vi "Control System.vi"(0 "VISA resource name":refnum<visa-resource-name>, 1 "Enable Zero Correct (F: Disable)":bool, 2 "Autoranging Speed (0: Fast)":i32(ring) items=["Fast", "Normal"], 5 "Enable Line Synchronization (T: Enable)":bool=TRUE, 7 "Enable A/D Hardware Limit (T: Enable)":bool=TRUE, 9 "Enable Humidity Readings (F: Disable)":bool, 11 "error in (no error)":errorcluster) -> (4 "VISA resource name out":refnum<visa-resource-name>, 15 "error out":errorcluster)   [LabVIEW 2019, in "Keithley 6517.lvlib"]
doc: "Controls the system line synchronization, A/D hardware limit, humidity readings, zero correction and autoranging.\n\nNote:\nRequires a separate scanner card. According to the manual 6521 or 6522, 7001 and 7002 can be used with this model. If the scanner card is not used the error -241, \"Hardware missing\" will be generated.\n\nThis VI is <B>NOT</B> compatible with model <B>6514</B>."
uses:
  Keithley 6517.lvlib
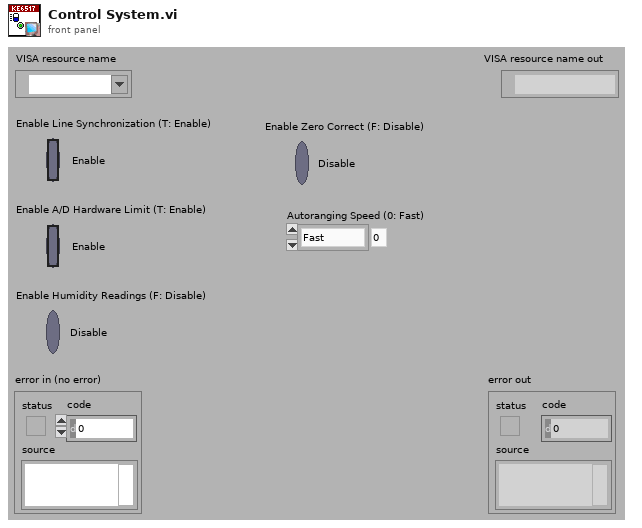
[diagram p1: front panel]
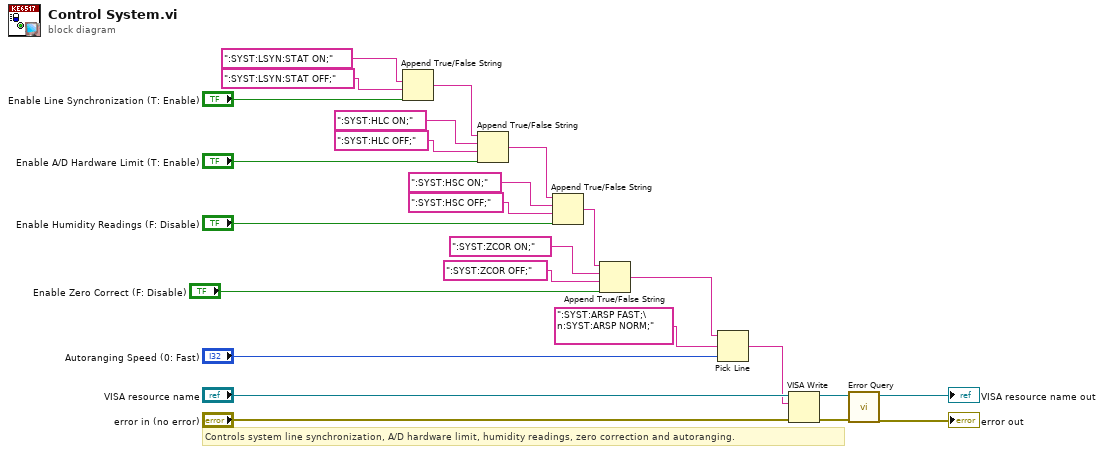
[diagram p0: block diagram]
diagram:
  # "Controls system line synchronization, A/D hardware limit, humidity readings, zero correction and autoranging."
  n1 = Append True/False String(1:"Enable Line Synchronization (T: Enable)", 2:":SYST:LSYN:STAT OFF;", 3:":SYST:LSYN:STAT ON;") -> (0:w22:string)  [unwired: 1 in]
  n2 = Append True/False String(1:"Enable A/D Hardware Limit (T: Enable)", 2:":SYST:HLC OFF;", 3:":SYST:HLC ON;", 4:w22) -> (0:w18:string)
  n3 = Append True/False String(1:"Enable Humidity Readings (F: Disable)", 2:":SYST:HSC OFF;", 3:":SYST:HSC ON;", 4:w18) -> (0:w2:string)
  n4 = Append True/False String(1:"Enable Zero Correct (F: Disable)", 2:":SYST:ZCOR OFF;", 3:":SYST:ZCOR ON;", 4:w2) -> (0:w1:string)
  n5 = Pick Line(string ("")=w1, multi-line string=":SYST:ARSP FAST;\n:SYST:ARSP NORM;", line index="Autoranging Speed (0: Fast)") -> (output string=w6:string)
  n6 = VISA Write(VISA resource name="VISA resource name", write buffer=w6, error in (no error)="error in (no error)") -> (VISA resource name out=w12:refnum<visa-resource-name>, error out=w11:errorcluster)  [unwired: 1 out]
  n7 = call "Error Query.vi"("error in (no error)"=w11, "VISA resource name"=w12) -> ("error out"=→"error out":errorcluster, "VISA resource name out"=→"VISA resource name out":refnum<visa-resource-name>)  [unwired: 6 in, 2 out]
